vi "Constants.vi"() -> ()   [LabVIEW 2019, in "DeltaPSControl Shared.lvlib"]
doc: "Use this Global VI to access the GUIDs assigned to the page resources of the Custom Device."
uses:
  DeltaPSControl Shared.lvlib
panel:
  in  "Tab Control":enum32{"GUIDS", "Constants", "Properties"}(tab)
  in  "Sequences page":string="5cfa443f-4e58-4866-a6f4-b959386199b6"
  in  "Status page":string="e75353bd-ff68-4c19-b56a-7e874564a189"
  in  "Indicators page":string="5b739410-4c38-4322-88c6-31c37b7a745d"
  in  "Controls page":string="2ad02c65-8b59-4d5c-9cd0-6e2197e40fa1"
  in  "DeltaPSControl":string="a9757bbc-b63a-4950-8d5b-061fccb06955"
  in  "sequences list":string="sequences list"
  in  "Def Port":u16=8462
  in  "Port":string="Port"
  in  "IP Address":string="IP Address"
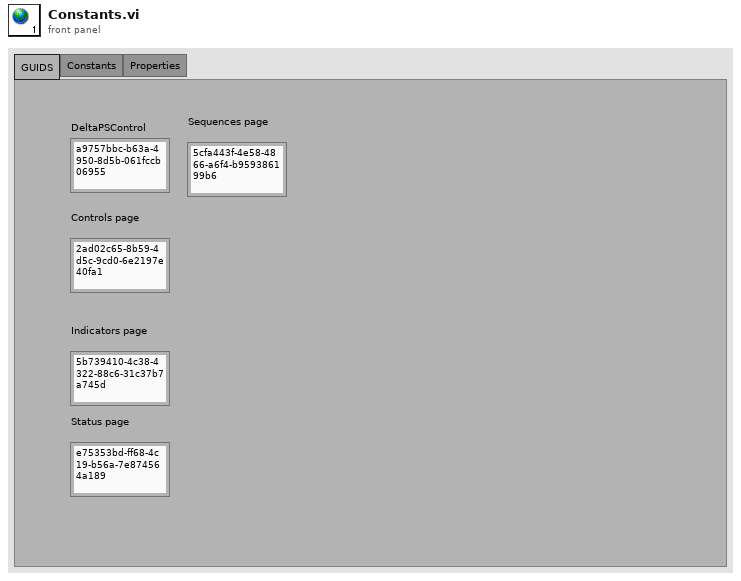
[diagram p1: front panel]
diagram:
